vi "MaxValue.vi"(8 "NewValue":dbl, 11 "CurrentMax":dbl) -> (2 "Max":dbl)   [LabVIEW 2016]
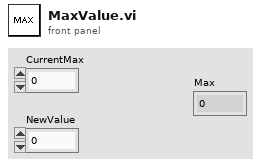
[diagram p1: front panel]
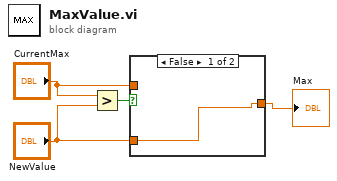
[diagram p0: block diagram]
diagram:
  n1 = Greater?(x="CurrentMax", y="NewValue") -> (0:w4:bool)
  n2 = case shown="False" w4 {
    tunnel: [w5 w6] -> w2
    tunnel: "CurrentMax" -> [_ w6]
    tunnel: "NewValue" -> [w5 _]
    frame False {
    }
    frame True {
    }
  }
  "Max" <- w2
